vi "VI.run_lua.vi"(5 "LuaVIEW reference":T1) -> (15 "error out":errorcluster)   [LabVIEW 2012]
doc: "Runs a VI asynchronously. This method maps to the LabVIEW run VI method.\nParameters:\nobj:self, object of VI to run.\n[bool:dispose_ref], Auto dispose reference, defaults to false when not specified. When true, the VI reference is passed to the run VI and will be cleaned up when that VI stops so that there is no more need to close the VI object after having called this method. It also prevents LabVIEW from wanting to save a template instance in development mode. Without this option, LabVIEW will pull the rug from under the run VI when the execution context that opened the VI object comes to a halt and the front panel of the run VI is not open even when the VI object is never closed.\nErrors:\nNot a VI object.\nDead VI object.\nVI is not in a runnable state."
uses:
  typedefs/t_LuaVIEW Reference.ctl
  subvis/private/LuaVIEW Pull (object).vi
  subvis/private/LuaVIEW Pull (boolean).vi
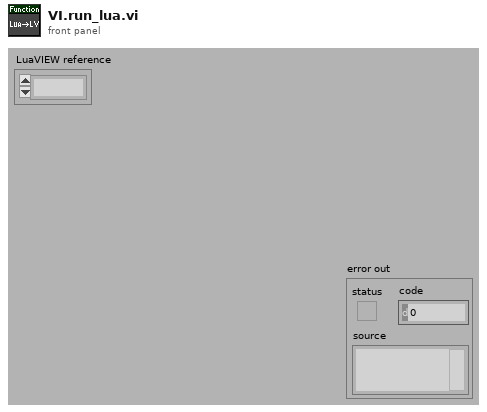
[diagram p1: front panel]
types:
  T1 = typedef "t_LuaVIEW Reference.ctl" = refnum<k1>
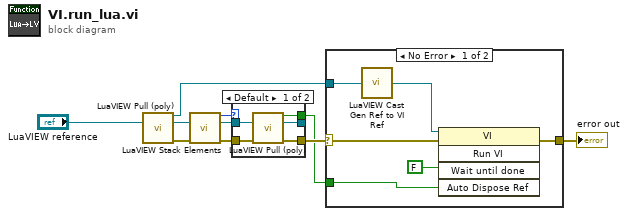
[diagram p0: block diagram]
diagram:
  n1 = call-poly "LuaVIEW Pull (poly).vi"("LuaVIEW reference in"="LuaVIEW reference") -> ("object refnum"=w1:refnum<vi>, "LuaVIEW reference out"=w4:T1, "error out"=w5:errorcluster)  [unwired: 11 in, 1 out]
  n2 = call "LuaVIEW Stack Elements.vi"("LuaVIEW reference in"=w4, "error in (no error)"=w5) -> ("elements"=w8:i32, "LuaVIEW reference out"=w6:T1, "error out"=w7:errorcluster)  [unwired: 11 in]
  n3 = case shown="Default" w8 {
    tunnel: w7 -> [w15 w16]
    tunnel: w6 -> [w14 w17]
    tunnel: [w13 w17] -> _
    tunnel: [w12 _] -> w2
    tunnel: [w11 w16] -> w3
    frame Default {
      n4 = call-poly "LuaVIEW Pull (poly).vi"("LuaVIEW reference in"=w14, "error in (no error)"=w15) -> ("boolean"=w12:bool, "LuaVIEW reference out"=w13:T1, "error out"=w11:errorcluster)  [unwired: 11 in]
    }
    frame 0 {
    }
  }
  n5 = case shown="No Error" w3 {
    selector: w3 -> [w23 w24]
    tunnel: [w21 w24] -> w9
    tunnel: w2 -> [w19 _]
    tunnel: w1 -> [w18 _]
    frame No Error {
      n6 = call "LuaVIEW Cast Gen Ref to VI Ref.vi"("refnum in"=w18) -> ("refnum out"=w22:refnum<vi>)  [unwired: 14 in]
      n7 = invoke class="VI" method="Run VI"(reference=w22, error in=w23, "Wait until done"=FALSE, "Auto Dispose Ref"=w19) -> (error out=w21:errorcluster)  [unwired: 1 in, 4 out]
    }
    frame Error {
    }
  }
  "error out" <- w9
